vi "Add BPP Data new1.vi"(8 "error in (no error)":errorcluster, 9 "Process Sub Step":string(combo), 10 "Records":T1, 11 "Test in":refnum<k24>) -> (0 "error out":errorcluster, 3 "Test out":refnum<k24>)   [LabVIEW 2018]
uses:
  C:/Program Files (x86)/National Instruments/LabVIEW 2018/user.lib/nEQdb_DLL/NEQdbAPI.dll
  Program Files (x86)/National Instruments/LabVIEW 2018/user.lib/nEQdb_DLL/NEQdbAPI.dll
  State data/Records.ctl
panel:
  in  "Enum":T2(ring)
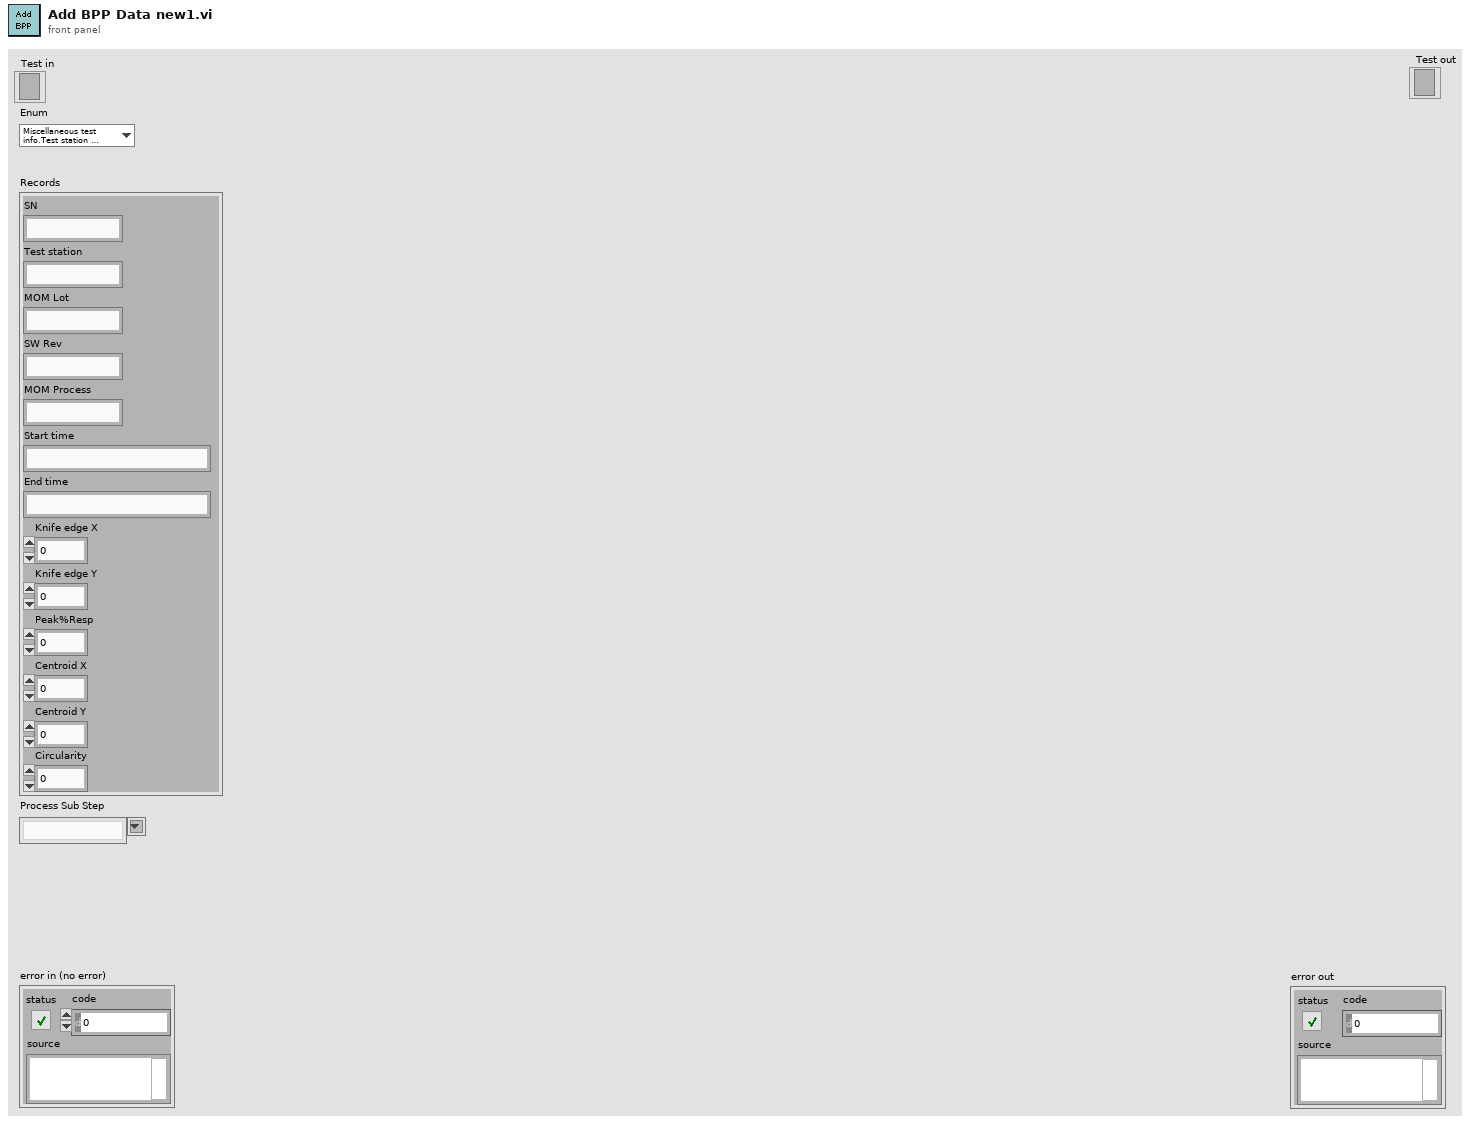
[diagram p1: front panel]
types:
  T1 = typedef "Records.ctl" = cluster{"SN":string, "Test station":string, "MOM Lot":string, "SW Rev":string, "MOM Process":string, "Start time":string, "End time":string, "Knife edge X":dbl, "Peak%Resp":dbl, "Centroid X":dbl, "Knife edge Y":dbl, "Centroid Y":dbl, "Circularity":dbl}
  T2 = enum16{"Miscellaneous test info.Test station number", "Miscellaneous test info.Software version", "MOM info.LotID", "MOM info.Process step name", "Process Sub Step", "BPP Test Results"}
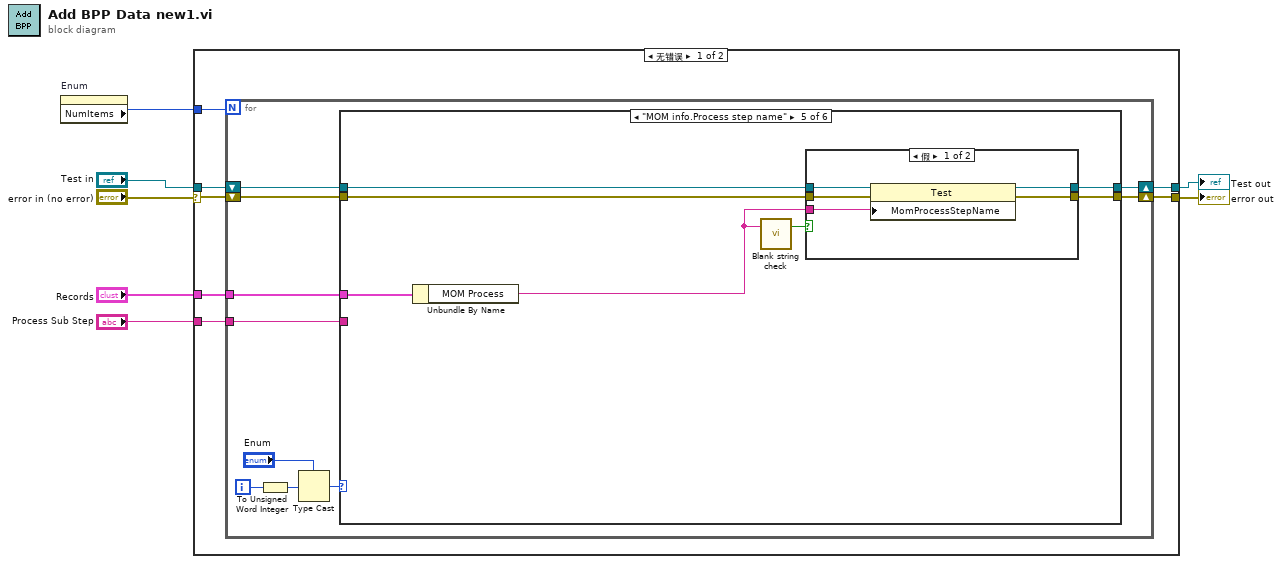
[diagram p0: block diagram]
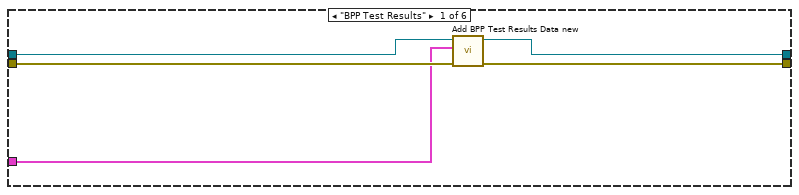
[diagram p2: hidden frame]
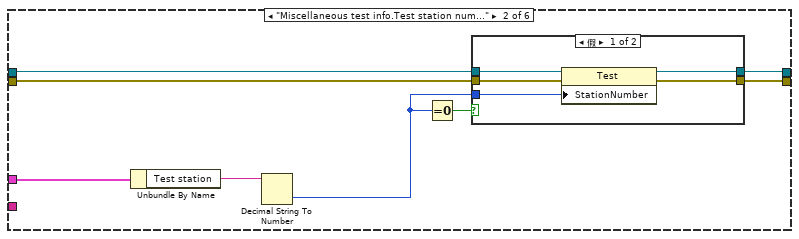
[diagram p3: hidden frame]
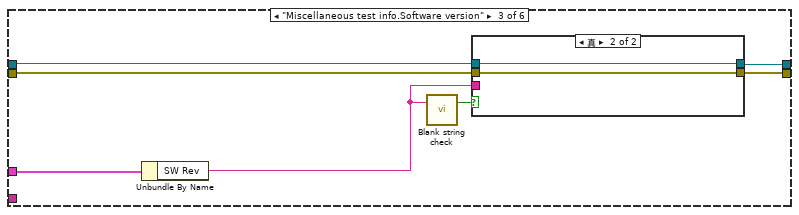
[diagram p5: hidden frame]
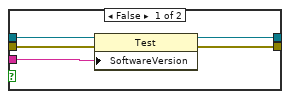
[diagram p6: hidden frame]
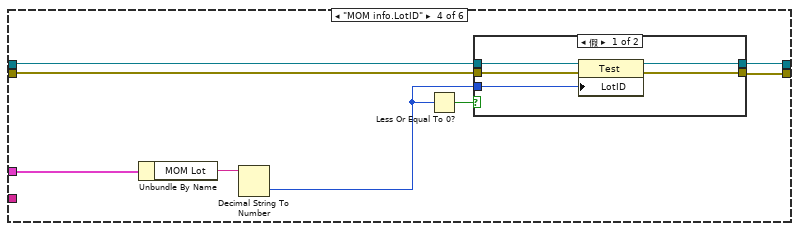
[diagram p7: hidden frame]
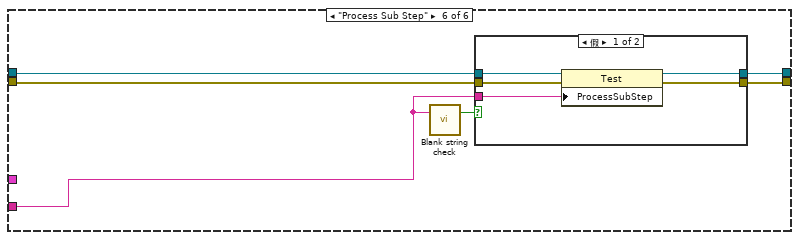
[diagram p10: hidden frame]
diagram:
  n1 = property on="Enum" class="Enum (严格)"() -> ("NumItems"=w6:u32)  [unwired: 2 in, 2 out]
  n2 = case shown="无错误" "error in (no error)" {
    selector: "error in (no error)" -> [w10 w101]
    tunnel: "Records" -> [w14 _]
    tunnel: "Test in" -> [w12 w102]
    tunnel: [w11 w102] -> w5
    tunnel: [w9 w101] -> w3
    tunnel: w6 -> [w13 _]
    tunnel: "Process Sub Step" -> [w8 _]
    frame No Error {
      n3 = for {
        N: w13 -> [_]
        shift-right: [w18] -> w9
        shift-left: w10 -> [w19]
        tunnel: w14 -> [w17]
        shift-right: [w16] -> w11
        shift-left: w12 -> [w20]
        tunnel: w8 -> [w15]
        i -> [w24]
        n4 = To Unsigned Word Integer(number=w24) -> (unsigned 16bit integer=w23:u16)
        n5 = Type Cast(type="Enum", x=w23) -> (*(type *) &x=w21:T2)
        n6 = case shown="\"MOM info.Process step name\"" w21 {
          tunnel: w20 -> [w29 w31 w49 w63 w78 w92]
          tunnel: w19 -> [w28 w30 w48 w62 w77 w91]
          tunnel: [w27 w32 w46 w60 w74 w90] -> w18
          tunnel: [w26 w33 w45 w61 w75 w89] -> w16
          tunnel: w17 -> [w25 w34 w47 w59 w76 _]
          tunnel: w15 -> [_ _ _ _ _ w88]
          frame "BPP Test Results" {
            n7 = call "Add BPP Test Results Data new.vi"("error in (no error)"=w28, "Collimation Data"=w25, "Test in"=w29) -> ("error out"=w27:errorcluster, "Test out"=w26:refnum<k24>)  [unwired: 7 in]
          }
          frame "Miscellaneous test info.Test station number" {
            n8 = Unbundle By Name(w34) -> ("Test station"=w36:string)
            n9 = Decimal String To Number(string=w36) -> (number=w35:i32)  [unwired: 2 in, 1 out]
            n10 = Equal To 0?(x=w35) -> (x = 0?=w37:bool)
            n11 = case shown="假" w37 {
              tunnel: w35 -> [w42 _]
              tunnel: w30 -> [w41 w43]
              tunnel: w31 -> [w40 w44]
              tunnel: [w39 w43] -> w32
              tunnel: [w38 w44] -> w33
              frame False {
                n12 = property class="Test"(reference=w40, error in=w41, "StationNumber"=w42) -> (reference out=w38:refnum<k24>, error out=w39:errorcluster)
              }
              frame True {
              }
            }
          }
          frame "Miscellaneous test info.Software version" {
            n13 = Unbundle By Name(w47) -> ("SW Rev"=w50:string)
            n14 = call <userlib>:"Blank string check.vi"("String for nEQdb"=w50) -> ("Blank or NaN?"=w51:bool)  [unwired: 2 in]
            n15 = case shown="真" w51 {
              tunnel: w50 -> [w56 _]
              tunnel: w48 -> [w55 w57]
              tunnel: w49 -> [w54 w58]
              tunnel: [w53 w57] -> w46
              tunnel: [w52 w58] -> w45
              frame False {
                n16 = property class="Test"(reference=w54, error in=w55, "SoftwareVersion"=w56) -> (reference out=w52:refnum<k24>, error out=w53:errorcluster)
              }
              frame True {
              }
            }
          }
          frame "MOM info.LotID" {
            n17 = Unbundle By Name(w59) -> ("MOM Lot"=w65:string)
            n18 = Decimal String To Number(string=w65) -> (number=w64:i32)  [unwired: 2 in, 1 out]
            n19 = Less Or Equal To 0?(x=w64) -> (x <= 0?=w66:bool)
            n20 = case shown="假" w66 {
              tunnel: w64 -> [w71 _]
              tunnel: w62 -> [w70 w72]
              tunnel: w63 -> [w69 w73]
              tunnel: [w68 w72] -> w60
              tunnel: [w67 w73] -> w61
              frame False {
                n21 = property class="Test"(reference=w69, error in=w70, "LotID"=w71) -> (reference out=w67:refnum<k24>, error out=w68:errorcluster)
              }
              frame True {
              }
            }
          }
          frame "MOM info.Process step name" {
            n22 = Unbundle By Name(w76) -> ("MOM Process"=w80:string)
            n23 = call <userlib>:"Blank string check.vi"("String for nEQdb"=w80) -> ("Blank or NaN?"=w79:bool)  [unwired: 2 in]
            n24 = case shown="假" w79 {
              tunnel: w77 -> [w85 w86]
              tunnel: w78 -> [w84 w87]
              tunnel: [w83 w86] -> w74
              tunnel: [w82 w87] -> w75
              tunnel: w80 -> [w81 _]
              frame False {
                n25 = property class="Test"(reference=w84, error in=w85, "MomProcessStepName"=w81) -> (reference out=w82:refnum<k24>, error out=w83:errorcluster)
              }
              frame True {
              }
            }
          }
          frame "Process Sub Step" {
            n26 = call <userlib>:"Blank string check.vi"("String for nEQdb"=w88) -> ("Blank or NaN?"=w93:bool)  [unwired: 2 in]
            n27 = case shown="假" w93 {
              tunnel: w91 -> [w98 w99]
              tunnel: w92 -> [w97 w100]
              tunnel: [w96 w99] -> w90
              tunnel: [w95 w100] -> w89
              tunnel: w88 -> [w94 _]
              frame False {
                n28 = property class="Test"(reference=w97, error in=w98, "ProcessSubStep"=w94) -> (reference out=w95:refnum<k24>, error out=w96:errorcluster)
              }
              frame True {
              }
            }
          }
        }
      }
    }
    frame Error {
    }
  }
  "Test out" <- w5
  "error out" <- w3
